vi "Example.vi"() -> ()   [LabVIEW 2020]
uses:
  Teaching View/Teaching View XControl.xctl
panel:
  in  "Initial Limit Position":cluster{"Lower Limit":dbl, "Upper Limit":dbl}={"Lower Limit"=4.0, "Upper Limit"=8.0}
  in  "Initial x-axis range":cluster{"Low Value":dbl, "High Value":dbl}={"Low Value"=0.0, "High Value"=10.0}
  in  "stop":bool
  out "Lower Limit":dbl
  out "Upper Limit":dbl
  in  "Teaching View XControl":T1(xcontrol)
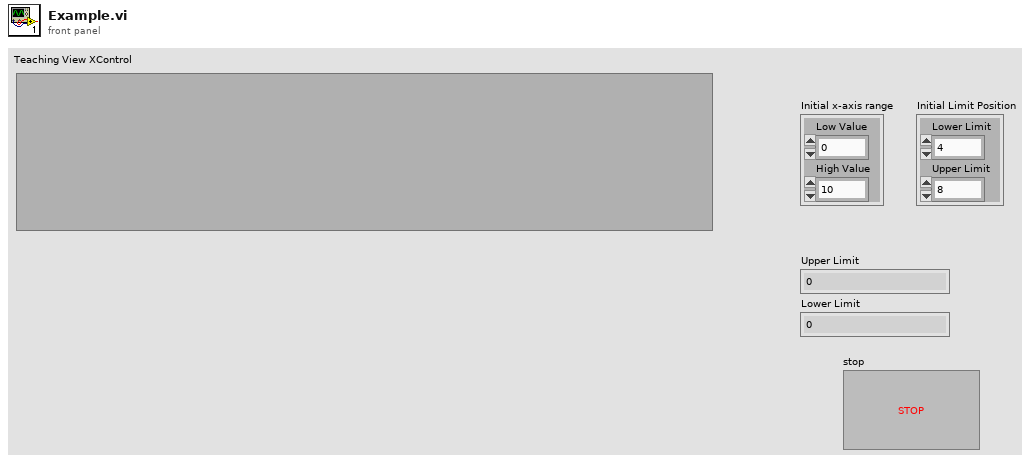
[diagram p1: front panel]
types:
  T1 = cluster{"Upper Limit":dbl, "Lower Limit":dbl, "Measure":dbl[]}
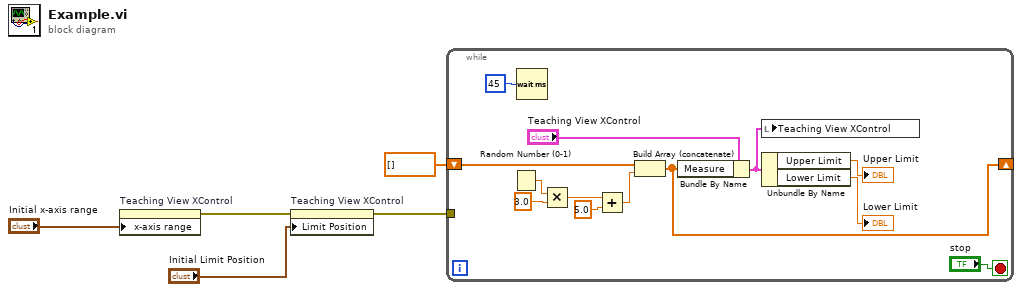
[diagram p0: block diagram]
diagram:
  n1 = property on="Teaching View XControl" class="Teaching View XControl (strict)"("x-axis range"="Initial x-axis range") -> (error out=w3:errorcluster)  [unwired: 2 in, 1 out]
  n2 = property on="Teaching View XControl" class="Teaching View XControl (strict)"(error in=w3, "Limit Position"="Initial Limit Position") -> (error out=w1:errorcluster)  [unwired: 1 in, 1 out]
  n3 = while {
    shift-right: [w6] -> _
    shift-left: dbl[] [] -> [w12]
    tunnel: w1 -> [_]
    stop <- "stop" stop-if-true
    n4 = Random Number (0-1)() -> (number: 0 to 1=w11:dbl)
    n5 = Wait (ms)(milliseconds to wait=u32 45) -> ()  [unwired: 1 out]
    n6 = Multiply(x=w11, y=3.0) -> (x*y=w9:dbl)
    n7 = Add(x=w9, y=5.0) -> (x+y=w7:dbl)
    n8 = Build Array (concatenate)(w12, w7) -> (w6:dbl[])
    n9 = Bundle By Name(cluster="Teaching View XControl", "Measure"=w6) -> (w15:T1)
    n10 = local write "Teaching View XControl"(w15) -> ()
    n11 = Unbundle By Name(w15) -> ("Upper Limit"=→"Upper Limit":dbl, "Lower Limit"=→"Lower Limit":dbl)
  }
